vi "Request Data JSON.vi"(8 "error in (no error)":errorcluster, 11 "SetInputMute in":refnum<class "SetInputMute.lvclass">) -> (0 "error out":errorcluster, 2 "Request Data JSON":string, 3 "SetInputMute out":refnum<class "SetInputMute.lvclass">)   [LabVIEW 2020, in "obs-websocket.lvlib" / "SetInputMute.lvclass"]
uses:
  SetInputMute.lvclass
  SetInputMute.lvclass/SetInputMute.ctl
  c595328c-9d07-4abc-969a-d70eb60fd32b.vi
  <vilib>/JDP Science/JSONtext/Variant to JSON Text.vi
  <vilib>/JDP Science/JSONtext/LVClass Serializer/JSONtext LVClass Serializer.lvclass
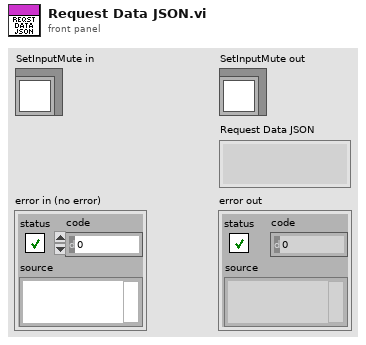
[diagram p1: front panel]
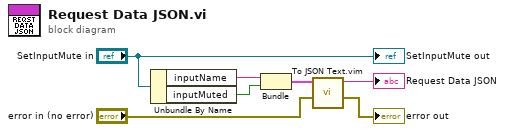
[diagram p0: block diagram]
diagram:
  n1 = Unbundle By Name("SetInputMute in") -> ("inputName"=w4:string, "inputMuted"=w3:bool)
  n2 = Bundle("inputName"=w4, "inputMuted"=w3) -> (w2:cluster{"inputName":string, "inputMuted":bool})  [unwired: 1 in]
  n3 = call "To JSON Text.vim"("error in (no error)"="error in (no error)", "Anything"=w2) -> ("error out"=→"error out":errorcluster, "<JSON>"=→"Request Data JSON":string)  [unwired: 8 in]
  "SetInputMute out" <- "SetInputMute in"
